vi "Append KLB File Name.vi"(8 "Iteration":i32, 11 "Path In":path) -> (3 "Path Out":path)   [LabVIEW 2013]
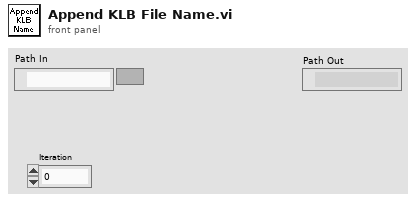
[diagram p1: front panel]
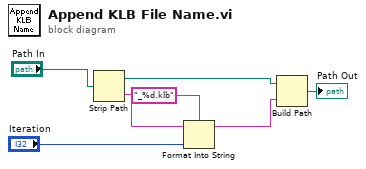
[diagram p0: block diagram]
diagram:
  n1 = Strip Path(path="Path In") -> (stripped path=w3:path, name=w6:string)
  n2 = Format Into String(format string="_%d.klb", initial string=w6, "Iteration") -> (resulting string=w2:string)  [unwired: 1 in, 1 out]
  n3 = Build Path(base path=w3, name or relative path=w2) -> (appended path=→"Path Out":path)
